vi "Main.vi"() -> ()   [LabVIEW 2013]
doc: "使用该模板构建简单状态机设计模式。各状态执行代码并决定转移状态。"
uses:
  C:/Program Files (x86)/MVS/Development/DotNet/AnyCpu/MvCamCtrl.Net.dll
  Program Files (x86)/MVS/Development/DotNet/AnyCpu/MvCamCtrl.Net.dll
  controls/RetureState.ctl
panel:
  out "DecodeParam":refnum<k24>
  out "PixelConvertParam":refnum<k24>
  out "HB_Decode":i32
  out "ConvertPixelType":i32
  out "FrameNum":u32 caption="帧号"
  out "ResultingFrameRate":sgl caption="采集帧率："
  out "Processed Frame":dbl caption="处理帧率："
  out "?":T1(plugin-control)
  in  "SetParam":bool
  in  "GetParam":bool caption="获取参数"
  out "error out":T2 caption="错误输出" {"code" format="%x"}
  out "CFrameoutEx":refnum<k24>
  out "PayloadSize":u32 caption="帧负载大小："
  out "CFloatValue":refnum<k24>
  out "CEnumValue":refnum<k24>
  out "CIntValue":refnum<k24>
  out "Width":u32 caption="图像宽："
  out "Height":u32 caption="图像高："
  in  "error in":errorcluster caption="错误输入" {"code" format="%x"}
  out "CCameraInfoList":refnum<k24>
  in  "PixelFormat":u32 caption="像素格式" format="%x"
  in  "Gain":sgl caption="增益(dB)" min=0 max=20 format="%.4f"
  in  "ExposureTime":sgl=5.0 caption="曝光时间(us)" min=5 max=100000 format="%.4f"
  in  "TriggerSoftWare":bool
  in  "AcquisitionStop":bool
  in  "TriggerMode":bool
  in  "Continuous":bool
  in  "AcquisitionStart":bool caption="开始采集"
  out "GrabbingStatus":bool caption="图像采集"
  out "OpenSatatus":bool caption="相机打开"
  in  "退出":bool
  in  "CloseDevice":bool
  in  "OpenDevice":bool
  in  "EumDevice":bool
  in  "DeviceList":u16(ring) caption="设备列表"
  out "DeviceNum":i32 caption="设备个数"
  out "CCamera":refnum<k24>
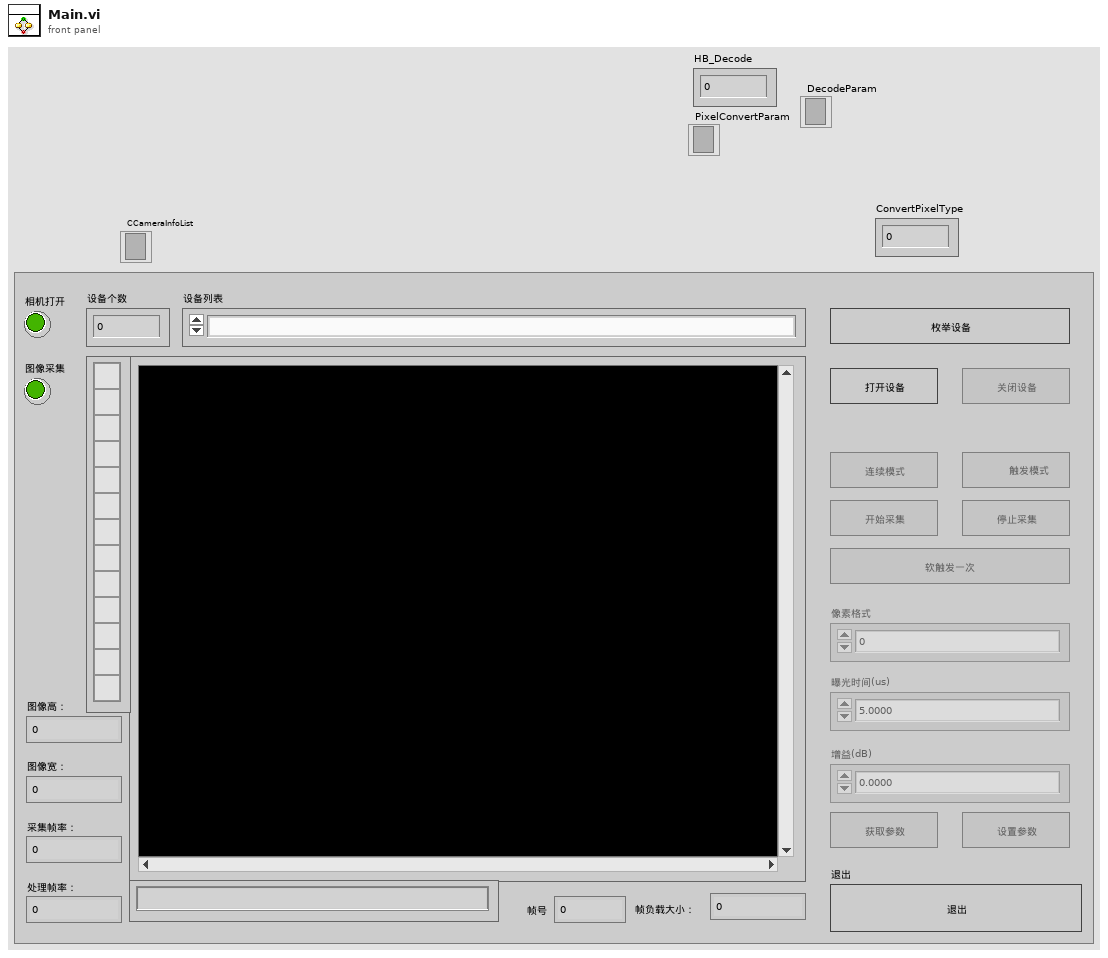
[diagram p1: front panel]
types:
  T1 = typedef "IMAQ Image.ctl" = refnum<image>
  T2 = typedef "RetureState.ctl" = errorcluster
  T3 = enum8{"Enabled", "Disabled", "Disabled and Grayed Out"}
  T4 = typedef "Image Type" = u32
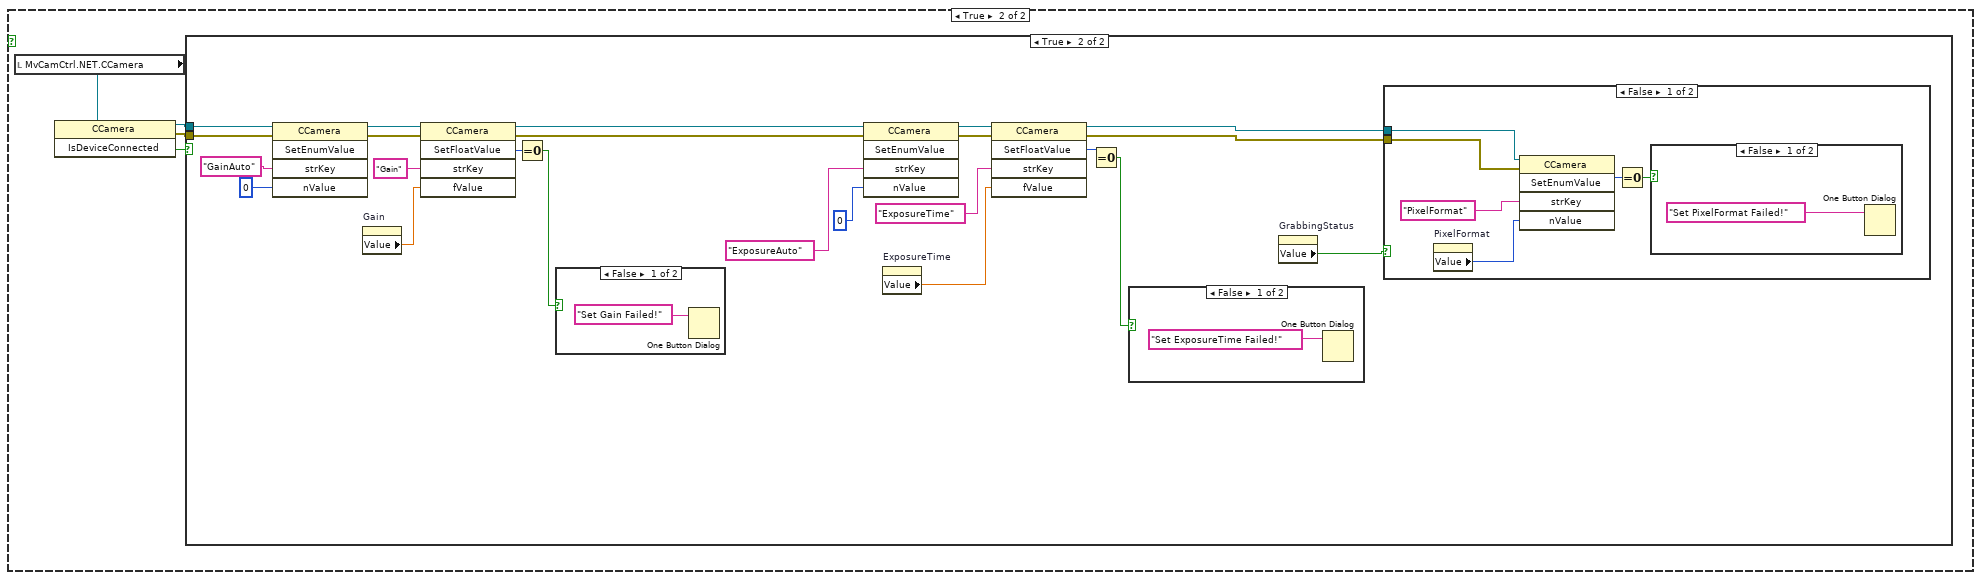
[diagram p4: hidden frame]
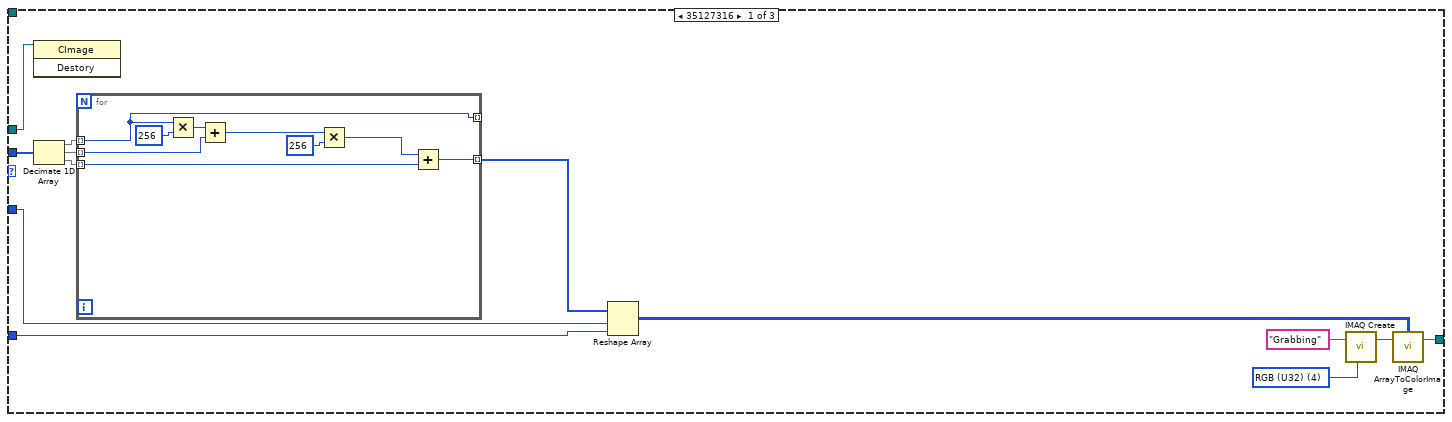
[diagram p15: hidden frame]
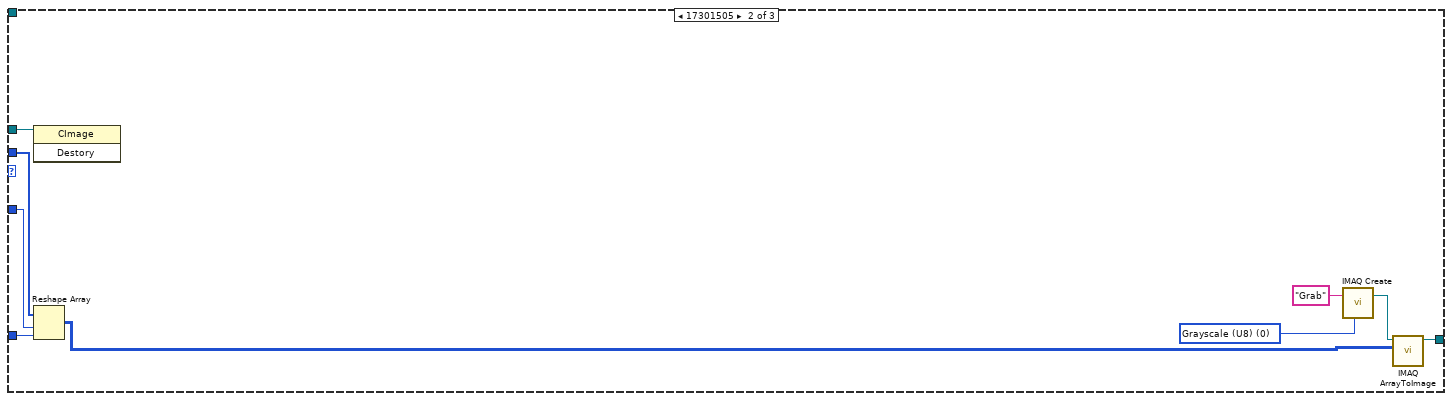
[diagram p16: hidden frame]
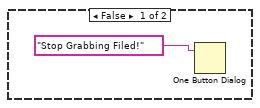
[diagram p19: hidden frame]
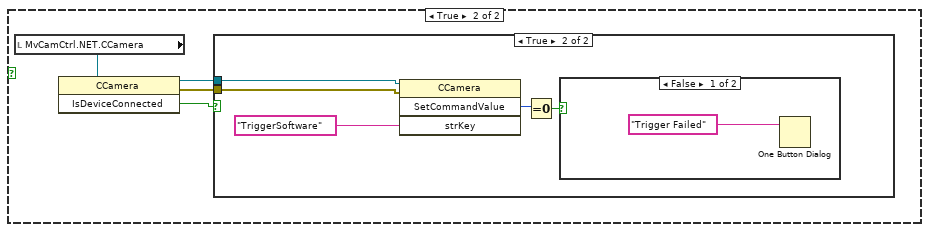
[diagram p20: hidden frame]
diagram:
  n1 = constructor class="CPixelConvertParam"() -> (reference out=→"PixelConvertParam":refnum<k24>)  [unwired: 3 in, 2 out]
  n2 = constructor class="CIntValue"() -> (reference out=→"CIntValue":refnum<k24>)  [unwired: 3 in, 2 out]
  n3 = constructor class="CEnumValue"() -> (reference out=→"CEnumValue":refnum<k24>)  [unwired: 3 in, 2 out]
  n4 = constructor class="CFloatValue"() -> (reference out=→"CFloatValue":refnum<k24>)  [unwired: 3 in, 2 out]
  n5 = constructor class="CCamera"() -> (reference out=→"CCamera":refnum<k24>)  [unwired: 3 in, 2 out]
  n6 = constructor class="CDecodeParam"() -> (reference out=→"DecodeParam":refnum<k24>)  [unwired: 3 in, 2 out]
  n7 = constructor class="CFrameoutEx"() -> (reference out=→"CFrameoutEx":refnum<k24>)  [unwired: 3 in, 2 out]
  n8 = while {
    tunnel: ["退出"] -> w9
    tunnel: "error in" -> [w15]
    stop <- "退出" stop-if-true
    n9 = property on="GrabbingStatus" class="Bool (strict)"() -> ("Value"=w14:bool)  [unwired: 2 in, 2 out]
    n10 = case shown="True" "GetParam" {
      frame False {
      }
      frame True {
        n11 = local read "CCamera"() -> (w63:refnum<k24>)
        n12 = invoke class="CCamera" method="IsDeviceConnected"(reference=w63) -> (reference out=w61:refnum<k24>, error out=w60:errorcluster, "IsDeviceConnected"=w62:bool)  [unwired: 2 in]
        n13 = case shown="True" w62 {
          tunnel: w61 -> [_ w73]
          tunnel: w60 -> [_ w72]
          frame False {
          }
          frame True {
            n14 = local read "CEnumValue"() -> (w74:refnum<k24>)
            n15 = invoke on="调用节点" class="CCamera" method="GetEnumValue"(reference=w73, error in=w72, "strKey"="PixelFormat", "oValue"=w74) -> (reference out=w80:refnum<k24>, error out=w77:errorcluster, "oValue"=w81:refnum<k24>)  [unwired: 1 in, 2 out]
            n16 = property on="属性节点" class="CEnumValue"(reference=w81) -> ("CurValue"=w82:u32)  [unwired: 1 in, 2 out]
            n17 = local read "CFloatValue"() -> (w71:refnum<k24>)
            n18 = property on="PixelFormat" class="DigNum (strict)"("Value"=w82) -> ()  [unwired: 2 in, 2 out]
            n19 = invoke on="调用节点" class="CCamera" method="GetFloatValue"(reference=w80, error in=w77, "strKey"="ExposureTime", "oValue"=w71) -> (reference out=w79:refnum<k24>, error out=w76:errorcluster, "oValue"=w65:refnum<k24>)  [unwired: 1 in, 2 out]
            n20 = property on="属性节点" class="CFloatValue"(reference=w65) -> ("CurValue"=w64:sgl)  [unwired: 1 in, 2 out]
            n21 = local read "CFloatValue"() -> (w68:refnum<k24>)
            n22 = property on="ExposureTime" class="DigNum (strict)"("Value"=w64) -> ()  [unwired: 2 in, 2 out]
            n23 = invoke on="调用节点" class="CCamera" method="GetFloatValue"(reference=w79, error in=w76, "strKey"="Gain", "oValue"=w68) -> ("oValue"=w78:refnum<k24>)  [unwired: 1 in, 4 out]
            n24 = property on="属性节点" class="CFloatValue"(reference=w78) -> (error out=w67:errorcluster, "CurValue"=w66:sgl)  [unwired: 1 in, 1 out]
            n25 = property on="Gain" class="DigNum (strict)"(error in=w67, "Value"=w66) -> ()  [unwired: 1 in, 2 out]
          }
        }
      }
    }
    n26 = case shown="False" "TriggerMode" {
      frame False {
      }
      frame True {
        n27 = local read "CCamera"() -> (w249:refnum<k24>)
        n28 = property class="MV_CAM_TRIGGER_MODE"() -> ("MV_TRIGGER_MODE_ON"=w248:i32)  [unwired: 2 in, 2 out]
        n29 = invoke class="CCamera" method="SetEnumValue"(reference=w249, "strKey"="TriggerMode", "nValue"=w248) -> (reference out=w247:refnum<k24>, error out=w246:errorcluster, "SetEnumValue"=w244:i32)  [unwired: 2 in, 2 out]
        n30 = Equal To 0?(x=w244) -> (x = 0?=w245:bool)
        n31 = case shown="True" w245 {
          tunnel: w247 -> [_ w260]
          tunnel: w246 -> [_ w259]
          frame False {
            n32 = One Button Dialog(message="Set TiggerMode Filed!") -> ()  [unwired: 1 in, 1 out]
          }
          frame True {
            n33 = property class="MV_CAM_TRIGGER_SOURCE"() -> ("MV_TRIGGER_SOURCE_SOFTWARE"=w252:i32)  [unwired: 2 in, 2 out]
            n34 = invoke class="CCamera" method="SetEnumValue"(reference=w260, error in=w259, "strKey"="TriggerSource", "nValue"=w252) -> (error out=w258:errorcluster)  [unwired: 1 in, 4 out]
            n35 = property on="Continuous" class="Bool"(error in=w258, "DisabledEnum"=T3."Enabled" ("禁用")) -> (error out=w257:errorcluster)  [unwired: 1 in, 1 out]
            n36 = property on="TriggerMode" class="Bool"(error in=w257, "DisabledEnum"=T3."Disabled and Grayed Out" ("禁用")) -> (error out=w256:errorcluster)  [unwired: 1 in, 1 out]
            n37 = property on="TriggerSoftWare" class="Bool"(error in=w256, "DisabledEnum"=T3."Enabled" ("禁用")) -> ()  [unwired: 1 in, 2 out]
          }
        }
      }
    }
    n38 = case shown="True" w14 {
      frame False {
      }
      frame True {
        n39 = local read "CCamera"() -> (w89:refnum<k24>)
        n40 = property on="PayloadSize" class="DigNum (strict)"() -> ("Value"=w84:u32)  [unwired: 2 in, 2 out]
        n41 = invoke class="CCamera" method="IsDeviceConnected"(reference=w89) -> (reference out=w87:refnum<k24>, error out=w86:errorcluster, "IsDeviceConnected"=w88:bool)  [unwired: 2 in]
        n42 = Initialize Array(0, w84) -> (w83:i32[])
        n43 = case shown="True" w88 {
          tunnel: w87 -> [_ w96]
          tunnel: w86 -> [_ w95]
          tunnel: w84 -> [_ w91]
          tunnel: w83 -> [_ w90]
          frame False {
          }
          frame True {
            n44 = local read "CFrameoutEx"() -> (w99:refnum<k24>)
            n45 = invoke class="CCamera" method="GetOneFrameTimeout"(reference=w96, error in=w95, "pData"=w90, "nDataSize"=w91, "pcFrameEx"=w99, "nMsec"=1000) -> (reference out=w94:refnum<k24>, error out=w98:errorcluster, "GetOneFrameTimeout"=w101:i32, "pData"=w97:u8[], "pcFrameEx"=w93:refnum<k24>)  [unwired: 1 in, 2 out]
            n46 = Equal To 0?(x=w101) -> (x = 0?=w100:bool)
            n47 = case shown="True" w100 {
              tunnel: w93 -> [_ w125]
              tunnel: w98 -> [_ w126]
              tunnel: w97 -> [_ w117]
              tunnel: w94 -> [_ w112]
              frame False {
              }
              frame True {
                n48 = property on="属性节点" class="CFrameoutEx"(reference=w125) -> ("pcImageInfoEx"=w124:refnum<k24>, "FrameSpec"=w122:refnum<k24>)  [unwired: 1 in, 2 out]
                n49 = property on="属性节点" class="CFrameSpecInfo"(reference=w122) -> ("FrameNum"=w121:u32)  [unwired: 1 in, 2 out]
                "FrameNum" <- w121
                n50 = property on="属性节点" class="CImageEx"(reference=w124) -> (error out=w102:errorcluster, "PixelType"=w106:i32, "Width"=w103:u16, "Height"=w104:u16, "FrameLen"=w105:u32)  [unwired: 1 in, 1 out]
                n51 = constructor class="CImage"(error in=w102, "pBufData"=w117, "enPixelType"=w106, "nFrameLen"=w105, "nHeight"=w104, "nWidth"=w103, "nHeightEx"=w104, "nWidthEx"=w103) -> (reference out=w116:refnum<k24>)  [unwired: 2 in, 9 out]
                n52 = call <vilib>:"Calculate Frames per Second.vi"("Update Interval (ms)"=1000, "Buffer Number"=w121) -> ("Processed Frames/s"=→"Processed Frame":dbl, "Acquired Frames/s"=→"ResultingFrameRate":dbl)  [unwired: 7 in, 1 out]
                n53 = property class="CImage"(reference=w116) -> (reference out=w114:refnum<k24>, "IsHBPixelType"=w115:bool)  [unwired: 1 in, 1 out]
                n54 = case shown="True" w115 {
                  tunnel: w114 -> [w191 w193]
                  tunnel: [w191 w197] -> w113
                  tunnel: w112 -> [_ w196]
                  frame False {
                  }
                  frame True {
                    n55 = local read "DecodeParam"() -> (w192:refnum<k24>)
                    n56 = property class="CDecodeParam" props=["InImage", "OutImage"](reference=w192, "InImage"=w193) -> (reference out=w194:refnum<k24>)  [unwired: 1 in, 2 out]
                    n57 = invoke class="CCamera" method="HB_Decode"(reference=w196, "pcDecodeParam"=w194) -> ("HB_Decode"=→"HB_Decode":i32, "pcDecodeParam"=w198:refnum<k24>)  [unwired: 2 in, 2 out]
                    n58 = property class="CDecodeParam" props=["OutImage", "FrameSpecInfo"](reference=w198) -> ("OutImage"=w197:refnum<k24>)  [unwired: 1 in, 3 out]
                  }
                }
                n59 = property class="CImage"(reference=w113) -> (reference out=w107:refnum<k24>, "ImageData"=w110:u8[], "PixelType"=w111:i32, "Width"=w109:u16, "Height"=w108:u16)  [unwired: 1 in, 1 out]
                n60 = case shown="Default" w111 {
                  tunnel: w110 -> [w135 w157 _]
                  tunnel: w126 -> [_ _ _]
                  tunnel: [w139 w152 w180] -> w123
                  tunnel: w112 -> [_ _ w171]
                  tunnel: w107 -> [w127 w149 w160]
                  tunnel: w109 -> [w129 w150 w167]
                  tunnel: w108 -> [w128 w151 w166]
                  frame 35127316 {
                    w137 = T4 4 items=["Grayscale (U8)", "Grayscale (I16)", "Grayscale (SGL)", "Complex (CSG)", "RGB (U32)", "HSL (U32)", "RGB (U64)", "Grayscale (U16)"] ("Image Type")
                    n61 = invoke class="CImage" method="Destory"(reference=w127) -> ()  [unwired: 2 in, 3 out]
                    n62 = Decimate 1D Array(w135) -> (w134:u8[], w133:u8[], w132:u8[])
                    n63 = for {
                      tunnel: [w140] -> _ mode=indexing
                      tunnel: w133 -> [w143] mode=indexing
                      tunnel: w132 -> [w142] mode=indexing
                      tunnel: [w141] -> w131 mode=indexing
                      tunnel: w134 -> [w140] mode=indexing
                      n64 = Multiply(x=w140, y=u16 256) -> (x*y=w147:u16)
                      n65 = Add(x=w147, y=w143) -> (x+y=w144:u16)
                      n66 = Multiply ("乘")(x=w144, y=u16 256) -> (x*y=w146:u32)
                      n67 = Add(x=w146, y=w142) -> (x+y=w141:u32)
                    }
                    n68 = Reshape Array(w131, w128, w129) -> (w130:u32[][])
                    n69 = call "IMAQ Create"("Image Name"="Grabbing", "Image Type"=w137) -> ("New Image"=w136:T1)  [unwired: 3 in, 1 out]
                    n70 = call "IMAQ ArrayToColorImage"("Image Pixels (U32)"=w130, "Image"=w136) -> ("Image Out"=w139:T1)  [unwired: 3 in, 1 out]
                  }
                  frame 17301505 {
                    w155 = T4 0 items=["Grayscale (U8)", "Grayscale (I16)", "Grayscale (SGL)", "Complex (CSG)", "RGB (U32)", "HSL (U32)", "RGB (U64)", "Grayscale (U16)"] ("Image Type")
                    n71 = invoke class="CImage" method="Destory"(reference=w149) -> ()  [unwired: 2 in, 3 out]
                    n72 = Reshape Array(w157, w151, w150) -> (w153:u8[][])
                    n73 = call "IMAQ Create"("Image Name"="Grab", "Image Type"=w155) -> ("New Image"=w154:T1)  [unwired: 3 in, 1 out]
                    n74 = call "IMAQ ArrayToImage"("Image Pixels (U8)"=w153, "Image"=w154) -> ("Image Out"=w152:T1)  [unwired: 8 in, 1 out]
                  }
                  frame Default {
                    w178 = T4 4 items=["Grayscale (U8)", "Grayscale (I16)", "Grayscale (SGL)", "Complex (CSG)", "RGB (U32)", "HSL (U32)", "RGB (U64)", "Grayscale (U16)"] ("Image Type")
                    n75 = local read "PixelConvertParam"() -> (w158:refnum<k24>)
                    n76 = property class="CPixelConvertParam"(reference=w158, "InImage"=w160) -> (reference out=w170:refnum<k24>, "OutImage"=w165:refnum<k24>)  [unwired: 1 in, 1 out]
                    n77 = property class="CImage"(reference=w165, "PixelType"=u32 35127316) -> (error out=w163:errorcluster)  [unwired: 1 in, 1 out]
                    n78 = invoke class="CCamera" method="ConvertPixelType"(reference=w171, error in=w163, "pcCvtParam"=w170) -> (error out=w159:errorcluster, "ConvertPixelType"=→"ConvertPixelType":i32, "pcCvtParam"=w169:refnum<k24>)  [unwired: 1 in, 1 out]
                    n79 = invoke class="CImage" method="Destory"(reference=w160, error in=w159) -> ()  [unwired: 1 in, 3 out]
                    n80 = property class="CPixelConvertParam"(reference=w169) -> ("OutImage"=w162:refnum<k24>)  [unwired: 1 in, 2 out]
                    n81 = property class="CImage"(reference=w162) -> (error out=w161:errorcluster, "ImageData"=w168:u8[])  [unwired: 1 in, 1 out]
                    n82 = invoke class="CImage" method="Destory"(reference=w162, error in=w161) -> ()  [unwired: 1 in, 3 out]
                    n83 = Decimate 1D Array(w168) -> (w175:u8[], w174:u8[], w173:u8[])
                    n84 = for {
                      tunnel: [w182] -> _ mode=indexing
                      tunnel: w174 -> [w185] mode=indexing
                      tunnel: w173 -> [w184] mode=indexing
                      tunnel: [w183] -> w176 mode=indexing
                      tunnel: w175 -> [w182] mode=indexing
                      n85 = Multiply(x=w182, y=u16 256) -> (x*y=w189:u16)
                      n86 = Add(x=w189, y=w185) -> (x+y=w186:u16)
                      n87 = Multiply ("乘")(x=w186, y=u16 256) -> (x*y=w188:u32)
                      n88 = Add(x=w188, y=w184) -> (x+y=w183:u32)
                    }
                    n89 = Reshape Array(w176, w166, w167) -> (w177:u32[][])
                    n90 = call "IMAQ Create"("Image Name"="Grabbing", "Image Type"=w178) -> ("New Image"=w181:T1)  [unwired: 3 in, 1 out]
                    n91 = call "IMAQ ArrayToColorImage"("Image Pixels (U32)"=w177, "Image"=w181) -> ("Image Out"=w180:T1)  [unwired: 3 in, 1 out]
                  }
                }
                "?" <- w123
                n92 = call "IMAQ Dispose"("Image"=w123) -> ()  [unwired: 5 in, 1 out]
              }
            }
          }
        }
      }
    }
    n93 = case shown="False" "CloseDevice" {
      frame False {
      }
      frame True {
        n94 = local read "CCamera"() -> (w475:refnum<k24>)
        n95 = invoke class="CCamera" method="IsDeviceConnected"(reference=w475) -> (reference out=w474:refnum<k24>, error out=w473:errorcluster, "IsDeviceConnected"=w472:bool)  [unwired: 2 in]
        n96 = case shown="True" w472 {
          tunnel: w474 -> [_ w481]
          tunnel: w473 -> [_ w480]
          frame False {
          }
          frame True {
            w479 = T3."Disabled and Grayed Out" ("禁用")
            n97 = invoke class="CCamera" method="CloseDevice"(reference=w481, error in=w480) -> (reference out=w505:refnum<k24>, error out=w504:errorcluster)  [unwired: 1 in, 1 out]
            n98 = invoke class="CCamera" method="DestroyHandle"(reference=w505, error in=w504) -> (error out=w503:errorcluster)  [unwired: 1 in, 2 out]
            n99 = property on="OpenDevice" class="Bool"(error in=w503, "DisabledEnum"=T3."Enabled" ("禁用")) -> (error out=w499:errorcluster)  [unwired: 1 in, 1 out]
            n100 = property on="CloseDevice" class="Bool"(error in=w499, "DisabledEnum"=T3."Disabled and Grayed Out" ("禁用")) -> (error out=w498:errorcluster)  [unwired: 1 in, 1 out]
            n101 = property on="Continuous" class="Bool"(error in=w498, "DisabledEnum"=T3."Disabled and Grayed Out" ("禁用")) -> (error out=w497:errorcluster)  [unwired: 1 in, 1 out]
            n102 = property on="TriggerMode" class="Bool"(error in=w497, "DisabledEnum"=T3."Disabled and Grayed Out" ("禁用")) -> (error out=w484:errorcluster)  [unwired: 1 in, 1 out]
            n103 = property on="AcquisitionStop" class="Bool"(error in=w484, "DisabledEnum"=T3."Disabled and Grayed Out" ("禁用")) -> (error out=w496:errorcluster)  [unwired: 1 in, 1 out]
            n104 = property on="AcquisitionStart" class="Bool"(error in=w496, "DisabledEnum"=T3."Disabled and Grayed Out" ("禁用")) -> (error out=w482:errorcluster)  [unwired: 1 in, 1 out]
            n105 = property on="TriggerSoftWare" class="Bool"(error in=w482, "DisabledEnum"=T3."Disabled and Grayed Out" ("禁用")) -> (error out=w486:errorcluster)  [unwired: 1 in, 1 out]
            n106 = property on="PixelFormat" class="DigNum (strict)"(error in=w486, "DisabledEnum"=T3."Disabled and Grayed Out" ("禁用")) -> (error out=w485:errorcluster)  [unwired: 1 in, 1 out]
            n107 = property on="Gain" class="DigNum (strict)"(error in=w485, "DisabledEnum"=T3."Disabled and Grayed Out" ("禁用")) -> (error out=w495:errorcluster)  [unwired: 1 in, 1 out]
            n108 = property on="ExposureTime" class="DigNum (strict)"(error in=w495, "DisabledEnum"=w479) -> (error out=w478:errorcluster)  [unwired: 1 in, 1 out]
            n109 = property on="GetParam" class="Bool"(error in=w478, "DisabledEnum"=w479) -> (error out=w477:errorcluster)  [unwired: 1 in, 1 out]
            n110 = property on="SetParam" class="Bool"(error in=w477, "DisabledEnum"=w479) -> (error out=w476:errorcluster)  [unwired: 1 in, 1 out]
            n111 = property on="OpenSatatus" class="Bool (strict)"(error in=w476, "Value"=FALSE) -> (error out=w487:errorcluster)  [unwired: 1 in, 1 out]
            n112 = property on="GrabbingStatus" class="Bool (strict)"(error in=w487, "Value"=FALSE) -> ()  [unwired: 1 in, 2 out]
          }
        }
      }
    }
    n113 = case shown="True" "AcquisitionStart" {
      frame False {
      }
      frame True {
        n114 = local read "CCamera"() -> (w263:refnum<k24>)
        n115 = invoke class="CCamera" method="IsDeviceConnected"(reference=w263) -> (reference out=w261:refnum<k24>, "IsDeviceConnected"=w262:bool)  [unwired: 2 in, 1 out]
        n116 = case shown="True" w262 {
          tunnel: w261 -> [_ w265]
          frame False {
          }
          frame True {
            n117 = local read "CIntValue"() -> (w276:refnum<k24>)
            n118 = invoke class="CCamera" method="GetIntValue"(reference=w265, "strKey"="PayloadSize", "oValue"=w276) -> (reference out=w271:refnum<k24>, error out=w269:errorcluster, "oValue"=w280:refnum<k24>)  [unwired: 2 in, 2 out]
            n119 = local read "CEnumValue"() -> (w274:refnum<k24>)
            n120 = property class="CIntValue"(reference=w280) -> ("CurValue"=w275:i64)  [unwired: 1 in, 2 out]
            n121 = invoke on="调用节点" class="CCamera" method="GetEnumValue"(reference=w271, error in=w269, "strKey"="PixelFormat", "oValue"=w274) -> (reference out=w270:refnum<k24>, error out=w268:errorcluster, "oValue"=w273:refnum<k24>)  [unwired: 1 in, 2 out]
            n122 = property on="PayloadSize" class="DigNum (strict)"("Value"=w275) -> ()  [unwired: 2 in, 2 out]
            n123 = property class="CEnumValue"(reference=w273) -> ("CurValue"=w272:u32)  [unwired: 1 in, 2 out]
            n124 = invoke class="CCamera" method="StartGrabbing"(reference=w270, error in=w268) -> (reference out=w278:refnum<k24>, error out=w277:errorcluster, "StartGrabbing"=w264:i32)  [unwired: 1 in]
            n125 = property on="PixelFormat" class="DigNum (strict)"("Value"=w272) -> ()  [unwired: 2 in, 2 out]
            n126 = Equal To 0?(x=w264) -> (x = 0?=w279:bool)
            n127 = case shown="True" w279 {
              tunnel: w278 -> [_ w307]
              tunnel: w277 -> [_ w304]
              frame False {
                n128 = One Button Dialog(message="Satrt Grabbing Failed") -> ()  [unwired: 1 in, 1 out]
              }
              frame True {
                n129 = local read "CIntValue"() -> (w285:refnum<k24>)
                n130 = invoke class="CCamera" method="GetIntValue"(reference=w307, error in=w304, "strKey"="Width", "oValue"=w285) -> (reference out=w306:refnum<k24>, error out=w305:errorcluster, "oValue"=w302:refnum<k24>)  [unwired: 1 in, 2 out]
                n131 = property class="CIntValue"(reference=w302) -> (error out=w303:errorcluster, "CurValue"=w301:i64)  [unwired: 1 in, 1 out]
                n132 = local read "CIntValue"() -> (w284:refnum<k24>)
                n133 = property on="Width" class="DigNum (strict)"(error in=w303, "Value"=w301) -> ()  [unwired: 1 in, 2 out]
                n134 = invoke class="CCamera" method="GetIntValue"(reference=w306, error in=w305, "strKey"="Height", "oValue"=w284) -> (error out=w287:errorcluster, "oValue"=w291:refnum<k24>)  [unwired: 1 in, 3 out]
                n135 = property class="CIntValue"(reference=w291) -> (error out=w300:errorcluster, "CurValue"=w299:i64)  [unwired: 1 in, 1 out]
                n136 = property on="Height" class="DigNum (strict)"(error in=w300, "Value"=w299) -> ()  [unwired: 1 in, 2 out]
                n137 = property on="AcquisitionStart" class="Bool"(error in=w287, "DisabledEnum"=T3."Disabled and Grayed Out" ("禁用")) -> (error out=w298:errorcluster)  [unwired: 1 in, 1 out]
                n138 = property on="AcquisitionStop" class="Bool"(error in=w298, "DisabledEnum"=T3."Enabled" ("禁用")) -> (error out=w290:errorcluster)  [unwired: 1 in, 1 out]
                n139 = property on="PixelFormat" class="DigNum (strict)"(error in=w290, "DisabledEnum"=T3."Disabled and Grayed Out" ("禁用")) -> (error out=w286:errorcluster)  [unwired: 1 in, 1 out]
                n140 = property on="Continuous" class="Bool"(error in=w286) -> (error out=w297:errorcluster, "DisabledEnum"=w292:T3)  [unwired: 1 in, 1 out]
                n141 = Equal To 0?(x=w292) -> (x = 0?=w293:bool)
                n142 = case shown="False" w293 {
                  tunnel: w297 -> [w309 w313]
                  tunnel: [w308 w312] -> w295
                  frame False {
                    n143 = property on="TriggerSoftWare" class="Bool"(error in=w309, "DisabledEnum"=T3."Disabled and Grayed Out" ("禁用")) -> (error out=w308:errorcluster)  [unwired: 1 in, 1 out]
                  }
                  frame True {
                    n144 = property on="TriggerSoftWare" class="Bool"(error in=w313, "DisabledEnum"=T3."Enabled" ("禁用")) -> (error out=w312:errorcluster)  [unwired: 1 in, 1 out]
                  }
                }
                n145 = property on="GrabbingStatus" class="Bool (strict)"(error in=w295, "Value"=TRUE) -> ()  [unwired: 1 in, 2 out]
              }
            }
          }
        }
      }
    }
    n146 = case shown="True" "EumDevice" {
      tunnel: w15 -> [w387 w394]
      tunnel: [w387 w391] -> w13
      frame False {
      }
      frame True {
        n147 = invoke on="调用节点" class="CSystem" method="EnumDevices"(error in=w394, "nType"=u32 5) -> (error out=w393:errorcluster, "EnumDevices"=w388:refnum<k24>)  [unwired: 2 in, 2 out]
        "CCameraInfoList" <- w388
        n148 = property on="属性节点" class="List`1[[MvCamCtrl.NET.CCameraIn"(reference=w388, error in=w393) -> (reference out=w390:refnum<k24>, error out=w392:errorcluster, "Count"=w395:i32)
        "DeviceNum" <- w395
        n149 = Greater Than 0?(x=w395) -> (x > 0?=w396:bool)
        n150 = case shown="True" w396 {
          tunnel: w395 -> [_ w406]
          tunnel: w390 -> [_ w405]
          tunnel: w392 -> [w397 w403]
          tunnel: [w397 w400] -> w391
          frame False {
            n151 = One Button Dialog(message="Not Found Devices!", button name ("OK")="Warning") -> ()  [unwired: 1 out]
          }
          frame True {
            n152 = for {
              N: w406 -> [_]
              tunnel: [w417] -> w404 mode=indexing
              tunnel: w405 -> [w412]
              tunnel: w403 -> [w411]
              tunnel: [w408] -> w402 mode=indexing
              tunnel: [w407] -> w401 mode=indexing
              i -> [w416]
              n153 = invoke class="List`1[[MvCamCtrl.NET.CCameraIn" method="get_Item"(reference=w412, error in=w411, "index"=w416) -> (error out=w410:errorcluster, "get_Item"=w413:refnum<k24>)  [unwired: 1 in, 2 out]
              n154 = property class="CCameraInfo"(reference=w413, error in=w410) -> (reference out=w414:refnum<k24>, error out=w409:errorcluster, "nTLayerType"=w415:u32)
              n155 = case shown="20" w415 {
                tunnel: ["UnsupportDev" w429 w433 w446 w466] -> w417
                tunnel: w414 -> [_ w425 w437 w450 w464]
                tunnel: w409 -> [w418 w423 w436 w449 w460]
                tunnel: [w418 w421 w434 w448 w462] -> w408
                tunnel: [w418 w420 w435 w447 w461] -> w407
                frame 0, Default {
                }
                frame 1 {
                  n156 = To More Specific Class(target class=refnum<k24> refnum ("CGigECameraInfo"), reference=w425, error in=w423) -> (specific class reference=w424:refnum<k24>, error out=w422:errorcluster)
                  n157 = property class="CGigECameraInfo"(reference=w424, error in=w422) -> (error out=w421:errorcluster, "chModelName"=w428:string)  [unwired: 1 out]
                  n158 = property class="CGigECameraInfo"(reference=w424, error in=w422) -> (error out=w420:errorcluster, "chSerialNumber"=w430:string)  [unwired: 1 out]
                  n159 = Concatenate Strings("[GigE]" ("字符串"), w428, "（" ("字符串"), w430, "）" ("字符串")) -> (w429:string)
                }
                frame 16 {
                  n160 = To More Specific Class(target class=refnum<k24> refnum ("CGigECameraInfo"), reference=w437, error in=w436) -> (specific class reference=w439:refnum<k24>, error out=w438:errorcluster)
                  n161 = property class="CGigECameraInfo"(reference=w439, error in=w438) -> (error out=w434:errorcluster, "chModelName"=w442:string)  [unwired: 1 out]
                  n162 = property class="CGigECameraInfo"(reference=w439, error in=w438) -> (error out=w435:errorcluster, "chSerialNumber"=w443:string)  [unwired: 1 out]
                  n163 = Concatenate Strings("[VirGigE]" ("字符串"), w442, "（" ("字符串"), w443, "）" ("字符串")) -> (w433:string)
                }
                frame 32 {
                  n164 = To More Specific Class(target class=refnum<k24> refnum ("CUSBCameraInfo"), reference=w450, error in=w449) -> (specific class reference=w452:refnum<k24>, error out=w451:errorcluster)
                  n165 = property class="CUSBCameraInfo"(reference=w452, error in=w451) -> (error out=w447:errorcluster, "chSerialNumber"=w456:string)  [unwired: 1 out]
                  n166 = property class="CUSBCameraInfo"(reference=w452, error in=w451) -> (error out=w448:errorcluster, "chModelName"=w455:string)  [unwired: 1 out]
                  n167 = Concatenate Strings("[VirU3V]" ("字符串"), w455, "（" ("字符串"), w456, "）" ("字符串")) -> (w446:string)
                }
                frame 4 {
                  n168 = To More Specific Class(target class=refnum<k24> refnum ("CUSBCameraInfo"), reference=w464, error in=w460) -> (specific class reference=w463:refnum<k24>, error out=w459:errorcluster)
                  n169 = property class="CUSBCameraInfo"(reference=w463, error in=w459) -> (error out=w461:errorcluster, "chSerialNumber"=w469:string)  [unwired: 1 out]
                  n170 = property class="CUSBCameraInfo"(reference=w463, error in=w459) -> (error out=w462:errorcluster, "chModelName"=w468:string)  [unwired: 1 out]
                  n171 = Concatenate Strings("[U3V]" ("字符串"), w468, "（" ("字符串"), w469, "）" ("字符串")) -> (w466:string)
                }
              }
            }
            n172 = property on="DeviceList" class="Ring (strict)"("Strings []"=w404) -> ()  [unwired: 2 in, 2 out]
            n173 = Merge Errors(w402, w401) -> (w400:errorcluster)
          }
        }
      }
    }
    "error out" <- w13
    n174 = case shown="True" "OpenDevice" {
      frame False {
      }
      frame True {
        n175 = property on="DeviceList" class="Ring (strict)"() -> ("DigDisp.Text"=w323:string)  [unwired: 2 in, 2 out]
        n176 = local read "CCameraInfoList"() -> (w314:refnum<k24>)
        n177 = Decimal String To Number(string=w323) -> (number=w322:i32)  [unwired: 2 in, 1 out]
        n178 = invoke class="List`1[[MvCamCtrl.NET.CCameraIn" method="get_Item"(reference=w314, "index"=w322) -> (error out=w321:errorcluster, "get_Item"=w320:refnum<k24>)  [unwired: 2 in, 2 out]
        n179 = local read "CCamera"() -> (w318:refnum<k24>)
        n180 = invoke class="CCamera" method="CreateHandle"(reference=w318, error in=w321, "pcDevInfo"=w320) -> (reference out=w319:refnum<k24>, error out=w317:errorcluster, "CreateHandle"=w316:i32)  [unwired: 1 in, 1 out]
        n181 = Equal To 0?(x=w316) -> (x = 0?=w315:bool)
        n182 = case shown="True" w315 {
          tunnel: w317 -> [_ w328]
          tunnel: w320 -> [_ w327]
          tunnel: w319 -> [_ w326]
          frame False {
            n183 = One Button Dialog(message="Create Camera Handle Failed!") -> ()  [unwired: 1 in, 1 out]
          }
          frame True {
            n184 = invoke class="CCamera" method="OpenDevice"(reference=w326, error in=w328, "nAccessMode"=1, "nSwitchoverKey"=0) -> (reference out=w330:refnum<k24>, error out=w329:errorcluster, "OpenDevice"=w325:i32)  [unwired: 1 in, 2 out]
            n185 = Equal To 0?(x=w325) -> (x = 0?=w333:bool)
            n186 = case shown="True" w333 {
              tunnel: w330 -> [w338 w372]
              tunnel: w329 -> [w337 w371]
              tunnel: w327 -> [_ w348]
              frame False {
                n187 = invoke class="CCamera" method="DestroyHandle"(reference=w338, error in=w337) -> (error out=w334:errorcluster)  [unwired: 1 in, 2 out]
                n188 = One Button Dialog(message="Open Failed") -> ()  [unwired: 1 in, 1 out]
                n189 = property on="OpenSatatus" class="Bool (strict)"(error in=w334, "Value"=FALSE) -> ()  [unwired: 1 in, 2 out]
              }
              frame True {
                w339 = T3."Enabled" ("禁用")
                n190 = property class="MV_CAM_TRIGGER_MODE"() -> ("MV_TRIGGER_MODE_OFF"=w365:i32)  [unwired: 2 in, 2 out]
                n191 = invoke class="CCamera" method="SetEnumValue"(reference=w372, error in=w371, "strKey"="TriggerMode", "nValue"=w365) -> (reference out=w367:refnum<k24>, error out=w366:errorcluster)  [unwired: 1 in, 3 out]
                n192 = property on="属性节点" class="CCameraInfo"(reference=w348) -> ("nTLayerType"=w370:u32)  [unwired: 1 in, 2 out]
                n193 = property class="MV_CAM_ACQUISITION_MODE"() -> ("MV_ACQ_MODE_CONTINUOUS"=w363:i32)  [unwired: 2 in, 2 out]
                n194 = property class="CSystem"() -> ("MV_GIGE_DEVICE"=w362:i32)  [unwired: 2 in, 2 out]
                n195 = invoke class="CCamera" method="SetEnumValue"(reference=w367, error in=w366, "strKey"="AcquisitionMode", "nValue"=w363) -> (reference out=w344:refnum<k24>, error out=w345:errorcluster)  [unwired: 1 in, 3 out]
                n196 = Equal?(x=w362, y=w370) -> (x = y?=w369:bool)
                n197 = case shown="False" w369 {
                  tunnel: w344 -> [_ w380]
                  tunnel: w345 -> [w373 w379]
                  tunnel: [w373 w374] -> w361
                  frame False {
                  }
                  frame True {
                    n198 = invoke class="CCamera" method="GIGE_GetOptimalPacketSize"(reference=w380, error in=w379) -> (reference out=w377:refnum<k24>, error out=w376:errorcluster, "GIGE_GetOptimalPacketSize"=w375:i32)  [unwired: 1 in]
                    n199 = Greater Than 0?(x=w375) -> (x > 0?=w378:bool)
                    n200 = case shown="True" w378 {
                      tunnel: w377 -> [_ w386]
                      tunnel: w376 -> [w381 w385]
                      tunnel: w375 -> [_ w383]
                      tunnel: [w381 w382] -> w374
                      frame False {
                      }
                      frame True {
                        n201 = invoke class="CCamera" method="SetIntValue"(reference=w386, error in=w385, "strKey"="GevSCPSPacketSize", "nValue"=w383) -> (error out=w382:errorcluster)  [unwired: 1 in, 4 out]
                      }
                    }
                  }
                }
                n202 = property on="CloseDevice" class="Bool"(error in=w361, "DisabledEnum"=T3."Enabled" ("禁用")) -> (error out=w357:errorcluster)  [unwired: 1 in, 1 out]
                n203 = property on="TriggerMode" class="Bool"(error in=w357, "DisabledEnum"=T3."Enabled" ("禁用")) -> (error out=w360:errorcluster)  [unwired: 1 in, 1 out]
                n204 = property on="Continuous" class="Bool"(error in=w360, "DisabledEnum"=T3."Disabled and Grayed Out" ("禁用")) -> (error out=w346:errorcluster)  [unwired: 1 in, 1 out]
                n205 = property on="ExposureTime" class="DigNum (strict)"(error in=w346, "DisabledEnum"=T3."Enabled" ("禁用")) -> (error out=w359:errorcluster)  [unwired: 1 in, 1 out]
                n206 = property on="Gain" class="DigNum (strict)"(error in=w359, "DisabledEnum"=T3."Enabled" ("禁用")) -> (error out=w358:errorcluster)  [unwired: 1 in, 1 out]
                n207 = property on="PixelFormat" class="DigNum (strict)"(error in=w358, "DisabledEnum"=T3."Enabled" ("禁用")) -> (error out=w350:errorcluster)  [unwired: 1 in, 1 out]
                n208 = property on="OpenDevice" class="Bool"(error in=w350, "DisabledEnum"=T3."Disabled and Grayed Out" ("禁用")) -> (error out=w347:errorcluster)  [unwired: 1 in, 1 out]
                n209 = property on="AcquisitionStart" class="Bool"(error in=w347, "DisabledEnum"=w339) -> (error out=w343:errorcluster)  [unwired: 1 in, 1 out]
                n210 = property on="GetParam" class="Bool"(error in=w343, "DisabledEnum"=w339) -> (error out=w342:errorcluster)  [unwired: 1 in, 1 out]
                n211 = property on="SetParam" class="Bool"(error in=w342, "DisabledEnum"=w339) -> (error out=w341:errorcluster)  [unwired: 1 in, 1 out]
                n212 = property on="OpenSatatus" class="Bool (strict)"(error in=w341, "Value"=TRUE ("布尔")) -> ()  [unwired: 1 in, 2 out]
              }
            }
          }
        }
      }
    }
    n213 = case shown="False" "Continuous" {
      frame False {
      }
      frame True {
        n214 = local read "CCamera"() -> (w236:refnum<k24>)
        n215 = property class="MV_CAM_TRIGGER_MODE"() -> ("MV_TRIGGER_MODE_OFF"=w235:i32)  [unwired: 2 in, 2 out]
        n216 = invoke class="CCamera" method="SetEnumValue"(reference=w236, "strKey"="TriggerMode", "nValue"=w235) -> (error out=w234:errorcluster, "SetEnumValue"=w233:i32)  [unwired: 2 in, 3 out]
        n217 = Equal To 0?(x=w233) -> (x = 0?=w232:bool)
        n218 = case shown="True" w232 {
          tunnel: w234 -> [_ w238]
          frame False {
          }
          frame True {
            n219 = property on="TriggerMode" class="Bool"(error in=w238, "DisabledEnum"=T3."Enabled" ("禁用")) -> (error out=w242:errorcluster)  [unwired: 1 in, 1 out]
            n220 = property on="Continuous" class="Bool"(error in=w242, "DisabledEnum"=T3."Disabled and Grayed Out" ("禁用")) -> (error out=w241:errorcluster)  [unwired: 1 in, 1 out]
            n221 = property on="TriggerSoftWare" class="Bool"(error in=w241, "DisabledEnum"=T3."Disabled and Grayed Out" ("禁用")) -> ()  [unwired: 1 in, 2 out]
          }
        }
      }
    }
    n222 = case shown="False" "SetParam" {
      frame False {
      }
      frame True {
        n223 = local read "CCamera"() -> (w27:refnum<k24>)
        n224 = invoke class="CCamera" method="IsDeviceConnected"(reference=w27) -> (reference out=w25:refnum<k24>, error out=w24:errorcluster, "IsDeviceConnected"=w26:bool)  [unwired: 2 in]
        n225 = case shown="True" w26 {
          tunnel: w25 -> [_ w42]
          tunnel: w24 -> [_ w41]
          frame False {
          }
          frame True {
            n226 = invoke on="调用节点" class="CCamera" method="SetEnumValue"(reference=w42, error in=w41, "strKey"="GainAuto", "nValue"=0) -> (reference out=w47:refnum<k24>, error out=w46:errorcluster)  [unwired: 1 in, 3 out]
            n227 = property on="Gain" class="DigNum (strict)"() -> ("Value"=w43:sgl)  [unwired: 2 in, 2 out]
            n228 = invoke on="调用节点" class="CCamera" method="SetFloatValue"(reference=w47, error in=w46, "strKey"="Gain", "fValue"=w43) -> (reference out=w32:refnum<k24>, error out=w29:errorcluster, "SetFloatValue"=w45:i32)  [unwired: 1 in, 2 out]
            n229 = Equal To 0?(x=w45) -> (x = 0?=w44:bool)
            n230 = case shown="False" w44 {
              frame False {
                n231 = One Button Dialog(message="Set Gain Failed!") -> ()  [unwired: 1 in, 1 out]
              }
              frame True {
              }
            }
            n232 = invoke on="调用节点" class="CCamera" method="SetEnumValue"(reference=w32, error in=w29, "strKey"="ExposureAuto", "nValue"=0) -> (reference out=w37:refnum<k24>, error out=w36:errorcluster)  [unwired: 1 in, 3 out]
            n233 = property on="ExposureTime" class="DigNum (strict)"() -> ("Value"=w28:sgl)  [unwired: 2 in, 2 out]
            n234 = invoke on="调用节点" class="CCamera" method="SetFloatValue"(reference=w37, error in=w36, "strKey"="ExposureTime", "fValue"=w28) -> (reference out=w31:refnum<k24>, error out=w30:errorcluster, "SetFloatValue"=w35:i32)  [unwired: 1 in, 2 out]
            n235 = Equal To 0?(x=w35) -> (x = 0?=w34:bool)
            n236 = case shown="False" w34 {
              frame False {
                n237 = One Button Dialog(message="Set ExposureTime Failed!") -> ()  [unwired: 1 in, 1 out]
              }
              frame True {
              }
            }
            n238 = property on="GrabbingStatus" class="Bool (strict)"() -> ("Value"=w33:bool)  [unwired: 2 in, 2 out]
            n239 = case shown="False" w33 {
              tunnel: w31 -> [w52 _]
              tunnel: w30 -> [w51 _]
              frame False {
                n240 = property on="PixelFormat" class="DigNum (strict)"() -> ("Value"=w53:u32)  [unwired: 2 in, 2 out]
                n241 = invoke on="调用节点" class="CCamera" method="SetEnumValue"(reference=w52, error in=w51, "strKey"="PixelFormat", "nValue"=w53) -> ("SetEnumValue"=w54:i32)  [unwired: 1 in, 4 out]
                n242 = Equal To 0?(x=w54) -> (x = 0?=w55:bool)
                n243 = case shown="False" w55 {
                  frame False {
                    n244 = One Button Dialog(message="Set PixelFormat Failed!") -> ()  [unwired: 1 in, 1 out]
                  }
                  frame True {
                  }
                }
              }
              frame True {
              }
            }
          }
        }
      }
    }
    n245 = case shown="False" "TriggerSoftWare" {
      frame False {
      }
      frame True {
        n246 = local read "CCamera"() -> (w223:refnum<k24>)
        n247 = invoke class="CCamera" method="IsDeviceConnected"(reference=w223) -> (reference out=w222:refnum<k24>, error out=w221:errorcluster, "IsDeviceConnected"=w220:bool)  [unwired: 2 in]
        n248 = case shown="True" w220 {
          tunnel: w222 -> [_ w226]
          tunnel: w221 -> [_ w225]
          frame False {
          }
          frame True {
            n249 = invoke class="CCamera" method="SetCommandValue"(reference=w226, error in=w225, "strKey"="TriggerSoftware") -> ("SetCommandValue"=w227:i32)  [unwired: 1 in, 3 out]
            n250 = Equal To 0?(x=w227) -> (x = 0?=w228:bool)
            n251 = case shown="False" w228 {
              frame False {
                n252 = One Button Dialog(message="Trigger Failed") -> ()  [unwired: 1 in, 1 out]
              }
              frame True {
                n253 = One Button Dialog(message="SoftWare Trigger Once Success!") -> ()  [unwired: 1 in, 1 out]
              }
            }
          }
        }
      }
    }
    n254 = case shown="True" "AcquisitionStop" {
      frame False {
      }
      frame True {
        n255 = local read "CCamera"() -> (w202:refnum<k24>)
        n256 = invoke class="CCamera" method="StopGrabbing"(reference=w202) -> (error out=w199:errorcluster, "StopGrabbing"=w200:i32)  [unwired: 2 in, 1 out]
        n257 = Equal To 0?(x=w200) -> (x = 0?=w201:bool)
        n258 = case shown="True" w201 {
          tunnel: w199 -> [_ w215]
          frame False {
            n259 = One Button Dialog(message="Stop Grabbing Filed!") -> ()  [unwired: 1 in, 1 out]
          }
          frame True {
            n260 = property on="GrabbingStatus" class="Bool (strict)"(error in=w215, "Value"=FALSE) -> (error out=w214:errorcluster)  [unwired: 1 in, 1 out]
            n261 = property on="AcquisitionStart" class="Bool"(error in=w214, "DisabledEnum"=T3."Enabled" ("禁用")) -> (error out=w218:errorcluster)  [unwired: 1 in, 1 out]
            n262 = property on="AcquisitionStop" class="Bool"(error in=w218, "DisabledEnum"=T3."Disabled and Grayed Out" ("禁用")) -> (error out=w219:errorcluster)  [unwired: 1 in, 1 out]
            n263 = property on="TriggerSoftWare" class="Bool"(error in=w219, "DisabledEnum"=T3."Disabled and Grayed Out" ("禁用")) -> (error out=w206:errorcluster)  [unwired: 1 in, 1 out]
            n264 = property on="PixelFormat" class="DigNum (strict)"(error in=w206, "DisabledEnum"=T3."Enabled" ("禁用")) -> (error out=w205:errorcluster)  [unwired: 1 in, 1 out]
            n265 = property on="Height" class="DigNum (strict)"(error in=w205, "DisabledEnum"=T3."Enabled" ("禁用")) -> (error out=w212:errorcluster)  [unwired: 1 in, 1 out]
            n266 = property on="PayloadSize" class="DigNum (strict)"(error in=w212, "DisabledEnum"=T3."Enabled" ("禁用")) -> (error out=w211:errorcluster)  [unwired: 1 in, 1 out]
            n267 = property on="Width" class="DigNum (strict)"(error in=w211, "DisabledEnum"=T3."Enabled" ("禁用")) -> ()  [unwired: 1 in, 2 out]
          }
        }
      }
    }
  }
  n268 = case shown="True" w9 {
    frame False {
    }
    frame True {
      w509 = T3."Disabled and Grayed Out" ("禁用")
      n269 = local read "CCamera"() -> (w514:refnum<k24>)
      n270 = invoke class="CCamera" method="IsDeviceConnected"(reference=w514) -> (reference out=w513:refnum<k24>, error out=w510:errorcluster, "IsDeviceConnected"=w512:bool)  [unwired: 2 in]
      n271 = property on="OpenSatatus" class="Bool (strict)"() -> ("Value"=w511:bool)  [unwired: 2 in, 2 out]
      n272 = Or(x=w512, y=w511) -> (x .or. y?=w515:bool)
      n273 = case shown="True" w515 {
        tunnel: w513 -> [_ w540]
        tunnel: w510 -> [_ w539]
        frame False {
        }
        frame True {
          n274 = invoke class="CCamera" method="CloseDevice"(reference=w540, error in=w539) -> (reference out=w542:refnum<k24>, error out=w541:errorcluster)  [unwired: 1 in, 1 out]
          n275 = invoke class="CCamera" method="DestroyHandle"(reference=w542, error in=w541) -> ()  [unwired: 1 in, 3 out]
        }
      }
      n276 = property on="OpenDevice" class="Bool"("DisabledEnum"=T3."Enabled" ("禁用")) -> (error out=w535:errorcluster)  [unwired: 2 in, 1 out]
      n277 = property on="CloseDevice" class="Bool"(error in=w535, "DisabledEnum"=T3."Disabled and Grayed Out" ("禁用")) -> (error out=w534:errorcluster)  [unwired: 1 in, 1 out]
      n278 = property on="TriggerSoftWare" class="Bool"(error in=w534, "DisabledEnum"=T3."Disabled and Grayed Out" ("禁用")) -> (error out=w533:errorcluster)  [unwired: 1 in, 1 out]
      n279 = property on="AcquisitionStart" class="Bool"(error in=w533, "DisabledEnum"=T3."Disabled and Grayed Out" ("禁用")) -> (error out=w532:errorcluster)  [unwired: 1 in, 1 out]
      n280 = property on="AcquisitionStop" class="Bool"(error in=w532, "DisabledEnum"=T3."Disabled and Grayed Out" ("禁用")) -> (error out=w531:errorcluster)  [unwired: 1 in, 1 out]
      n281 = property on="Continuous" class="Bool"(error in=w531, "DisabledEnum"=T3."Disabled and Grayed Out" ("禁用")) -> (error out=w530:errorcluster)  [unwired: 1 in, 1 out]
      n282 = property on="TriggerMode" class="Bool"(error in=w530, "DisabledEnum"=T3."Disabled and Grayed Out" ("禁用")) -> (error out=w529:errorcluster)  [unwired: 1 in, 1 out]
      n283 = property on="ExposureTime" class="DigNum (strict)"(error in=w529, "DisabledEnum"=T3."Disabled and Grayed Out" ("禁用")) -> (error out=w528:errorcluster)  [unwired: 1 in, 1 out]
      n284 = property on="Gain" class="DigNum (strict)"(error in=w528, "DisabledEnum"=T3."Disabled and Grayed Out" ("禁用")) -> (error out=w518:errorcluster)  [unwired: 1 in, 1 out]
      n285 = property on="PixelFormat" class="DigNum (strict)"(error in=w518, "DisabledEnum"=w509) -> (error out=w508:errorcluster)  [unwired: 1 in, 1 out]
      n286 = property on="GetParam" class="Bool"(error in=w508, "DisabledEnum"=w509) -> (error out=w507:errorcluster)  [unwired: 1 in, 1 out]
      n287 = property on="SetParam" class="Bool"(error in=w507, "DisabledEnum"=w509) -> (error out=w506:errorcluster)  [unwired: 1 in, 1 out]
      n288 = property on="OpenSatatus" class="Bool (strict)"(error in=w506, "Value"=FALSE) -> (error out=w538:errorcluster)  [unwired: 1 in, 1 out]
      n289 = property on="GrabbingStatus" class="Bool (strict)"(error in=w538, "Value"=FALSE) -> (error out=w517:errorcluster)  [unwired: 1 in, 1 out]
      n290 = property on="DeviceNum" class="DigNum (strict)"(error in=w517, "Value"=0) -> ()  [unwired: 1 in, 2 out]
    }
  }
